vi "VI Tree.vi"   [LabVIEW 2015, in "BK Precision 983X Series.lvlib"]
doc: "This is the instrument driver for the B&K Precision 983X AC power supplies. The VI Tree displays all the user-callable VIs of the instrument driver in an organized table."
uses:
  <instrlib>/BK Precision 983X Series/BK Precision 983X Series.lvlib
panel:
  # "(c) 2017 B&K Precision Corporation.  ALL RIGHTS RESERVED."
  # "SEE DIAGRAM\nFOR VI TREE."
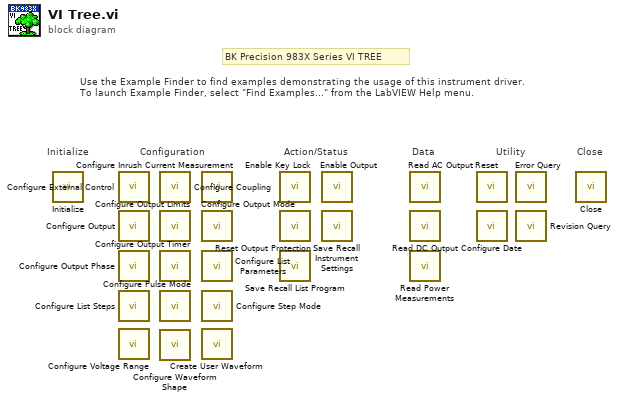
[diagram p0: block diagram]
diagram:
  # "BK Precision 983X Series VI TREE"
  # "Use the Example Finder to find examples demonstrating the usage of this instrument driver.\nTo launch Example Finder, select \"Find Examples...\" from the LabVIEW Help menu."
  # "Configuration"
  # "Utility"
  # "Data"
  # "Action/Status"
  # "Close"
  # "Initialize"
  n1 = call <instrlib>:"Initialize.vi"() -> ()  [unwired: 10 in, 2 out]
  n2 = call <instrlib>:"Configure External Control.vi"() -> ()  [unwired: 10 in, 2 out]
  n3 = call <instrlib>:"Configure Output.vi"() -> ()  [unwired: 10 in, 2 out]
  n4 = call <instrlib>:"Configure Output Phase.vi"() -> ()  [unwired: 10 in, 2 out]
  n5 = call <instrlib>:"Configure List Steps.vi"() -> ()  [unwired: 14 in, 2 out]
  n6 = call <instrlib>:"Configure Voltage Range.vi"() -> ()  [unwired: 10 in, 2 out]
  n7 = call <instrlib>:"Configure Coupling.vi"() -> ()  [unwired: 10 in, 2 out]
  n8 = call <instrlib>:"Configure Output Limits.vi"() -> ()  [unwired: 14 in, 2 out]
  n9 = call <instrlib>:"Configure Output Timer.vi"() -> ()  [unwired: 14 in, 2 out]
  n10 = call <instrlib>:"Configure Pulse Mode.vi"() -> ()  [unwired: 14 in, 2 out]
  n11 = call <instrlib>:"Configure Waveform Shape.vi"() -> ()  [unwired: 10 in, 2 out]
  n12 = call <instrlib>:"Configure Inrush Current Measurement.vi"() -> ()  [unwired: 10 in, 2 out]
  n13 = call <instrlib>:"Configure Output Mode.vi"() -> ()  [unwired: 10 in, 2 out]
  n14 = call <instrlib>:"Configure List Parameters.vi"() -> ()  [unwired: 14 in, 2 out]
  n15 = call <instrlib>:"Configure Step Mode.vi"() -> ()  [unwired: 14 in, 2 out]
  n16 = call <instrlib>:"Create User Waveform.vi"() -> ()  [unwired: 10 in, 2 out]
  n17 = call <instrlib>:"Enable Key Lock.vi"() -> ()  [unwired: 10 in, 2 out]
  n18 = call <instrlib>:"Reset Output Protection.vi"() -> ()  [unwired: 10 in, 2 out]
  n19 = call <instrlib>:"Save Recall List Program.vi"() -> ()  [unwired: 10 in, 2 out]
  n20 = call <instrlib>:"Enable Output.vi"() -> ()  [unwired: 10 in, 2 out]
  n21 = call <instrlib>:"Save Recall Instrument Settings.vi"() -> ()  [unwired: 10 in, 2 out]
  n22 = call <instrlib>:"Read AC Output.vi"() -> ()  [unwired: 7 in, 5 out]
  n23 = call <instrlib>:"Read DC Output.vi"() -> ()  [unwired: 8 in, 4 out]
  n24 = call <instrlib>:"Read Power Measurements.vi"() -> ()  [unwired: 7 in, 9 out]
  n25 = call <instrlib>:"Reset.vi"() -> ()  [unwired: 10 in, 2 out]
  n26 = call <instrlib>:"Configure Date.vi"() -> ()  [unwired: 10 in, 2 out]
  n27 = call <instrlib>:"Error Query.vi"() -> ()  [unwired: 8 in, 4 out]
  n28 = call <instrlib>:"Revision Query.vi"() -> ()  [unwired: 8 in, 4 out]
  n29 = call <instrlib>:"Close.vi"() -> ()  [unwired: 11 in, 1 out]
